vi "InitDVR.vi"(11 "DVR":T1) -> (2 "error out":errorcluster, 3 "DVR":T1)   [LabVIEW 2019, in "RemoteControl.ZMQ.lvlib" / "ZMQ.ContextManager.lvlib"]
uses:
  ZMQ.ContextManager.lvlib
  Context--DVR.ctl
  Context--Cluster.ctl
  <vilib>/addons/zeromq/zmq_context.lvclass
panel:
  out "Ref":u32
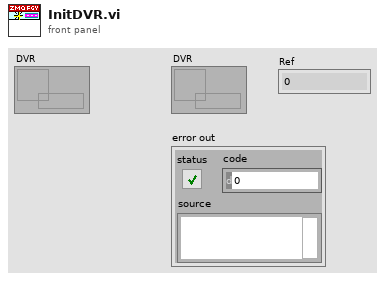
[diagram p1: front panel]
types:
  T1 = typedef "RemoteControl.ZMQ.lvlib/ZMQ.ContextManager.lvlib/Context--DVR.ctl" = refnum<data-value>
  T2 = typedef "RemoteControl.ZMQ.lvlib/ZMQ.ContextManager.lvlib/Context--Cluster.ctl" = cluster{"context":refnum<class "zmq_context.lvclass">, "counter":u32}
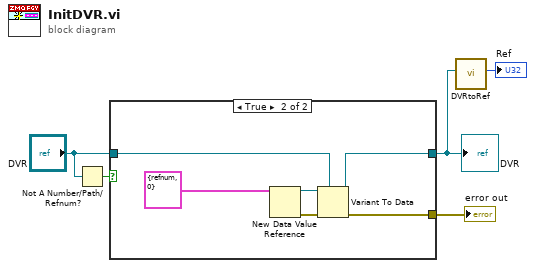
[diagram p0: block diagram]
diagram:
  n1 = Not A Number/Path/Refnum?(number/path/refnum="DVR") -> (NaN/Path/Refnum?=w4:bool)
  n2 = case shown="True" w4 {
    tunnel: [w6 w9] -> w2
    tunnel: "DVR" -> [w6 w12]
    tunnel: [_ w8] -> w3
    frame False {
    }
    frame True {
      n3 = New Data Value Reference(data value=T2 {"context"=refnum, "counter"=0} ("input cluster")) -> (data value reference=w10:refnum<data-value>, error out=w11:errorcluster)  [unwired: 1 in]
      n4 = Variant To Data(error in=w11, type=w12, Variant=w10) -> (data=w9:T1, error out=w8:errorcluster)
    }
  }
  "error out" <- w3
  "DVR" <- w2
  n5 = call "DVRtoRef.vi"("DVR"=w2) -> ("Ref"=→"Ref":u32)  [unwired: 10 in]
